vi "Read Measurement type.vi"(8 "error in (no error)":errorcluster, 11 "HC-Main in":refnum<class "HC-Main.lvclass">) -> (0 "error out":errorcluster, 2 "Measurement type":T1, 3 "HC-Main out":refnum<class "HC-Main.lvclass">)   [LabVIEW 2013, in "HardwareCharacterization.lvlib" / "HC-Main.lvclass"]
uses:
  HC-Main.lvclass
  Measurement-types.ctl
  HC-Main.lvclass/HC-Main.ctl
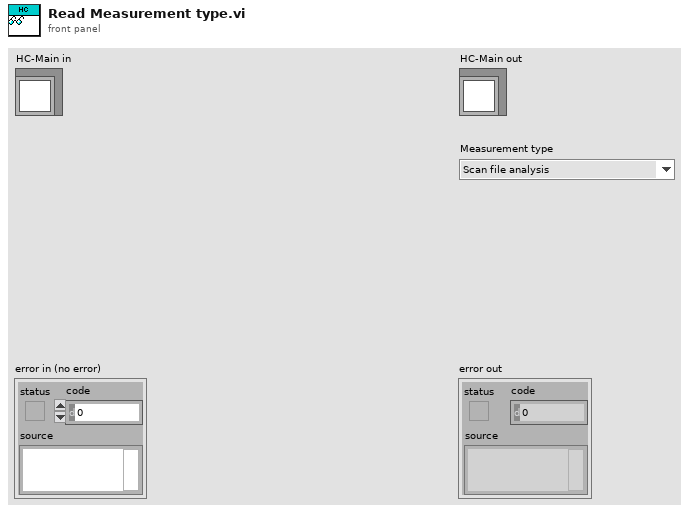
[diagram p1: front panel]
types:
  T1 = typedef "HardwareCharacterization.lvlib/HC-Main.lvclass/Measurement-types.ctl" = enum16{"Scan file analysis", "SM1000 position conversion", "SM1000 modulation timing", "Laser output response"}
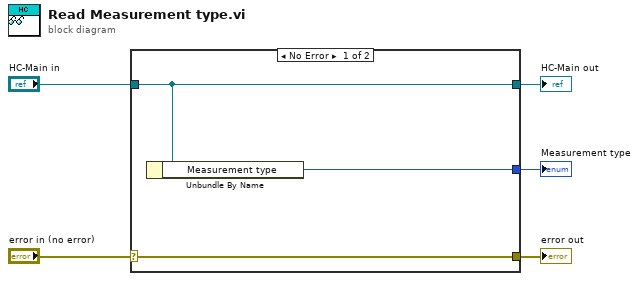
[diagram p0: block diagram]
diagram:
  n1 = case shown="No Error" "error in (no error)" {
    selector: "error in (no error)" -> [w8 w9]
    tunnel: [w8 w9] -> w4
    tunnel: [w7 w10] -> w2
    tunnel: "HC-Main in" -> [w7 w10]
    tunnel: [w6 _] -> w1
    frame No Error {
      n2 = Unbundle By Name(w7) -> ("Measurement type"=w6:T1)
    }
    frame Error {
    }
  }
  "error out" <- w4
  "HC-Main out" <- w2
  "Measurement type" <- w1
